vi "RxPkt - Init Packet Page.vi"(7 "Rx Section Cluster In":T2, 8 "error in (no error)":errorcluster, 11 "Node Ptr In":T1 format="%.0x") -> (0 "error out":errorcluster, 3 "Node Ptr Out":T1 format="%.0x", 5 "Rx Section Cluster Out":T2)   [LabVIEW 2016, in "UDP-Custom-Device System Explorer.lvlib"]
uses:
  UDP-Custom-Device System Explorer.lvlib
  Types/Page References/Refs - Rx Packets Page.ctl
  <vilib>/NI Veristand/Custom Device API/Custom Device Item Ref.ctl
  <vilib>/NI VeriStand/Custom Device API/Custom Device API.lvlib
  Property Accessors/Shared Packet Accessors.lvlib
  Property Accessors/Rx Channel Section Accessors.lvlib
  Property Accessors/Rx Packet Accessors.lvlib
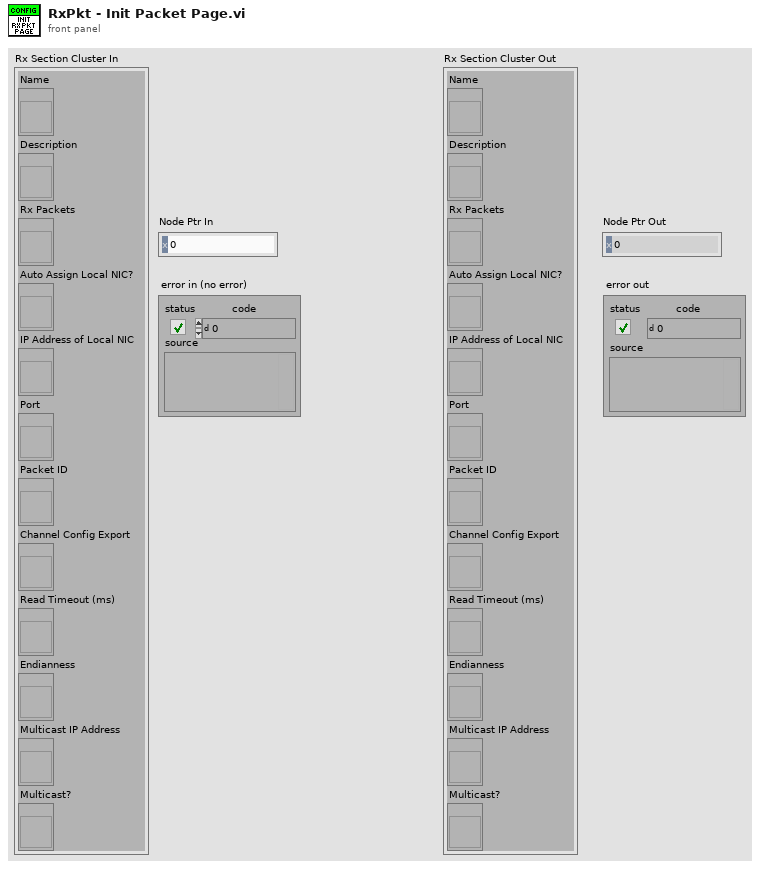
[diagram p1: front panel]
types:
  T1 = typedef "Custom Device API.lvlib/Custom Device Item Ref.ctl" = u64
  T2 = typedef "UDP-Custom-Device System Explorer.lvlib/Refs - Rx Packets Page.ctl" = cluster{"Name":refnum<vi>, "Description":refnum<vi>, "Rx Packets":refnum<vi>, "Auto Assign Local NIC?":refnum<vi>, "IP Address of Local NIC":refnum<vi>, "Port":refnum<vi>, "Packet ID":refnum<vi>, "Channel Config Export":refnum<vi>, "Read Timeout (ms)":refnum<vi>, "Endianness":refnum<vi>, "Multicast IP Address":refnum<vi>, "Multicast?":refnum<vi>}
  T3 = enum8{"Enabled", "Disabled", "Disabled and Grayed Out"}
  T4 = typedef "Custom Device API.lvlib/Custom Device Item Info.ctl" = cluster{"Name":string, "Is Channel":bool, "GUID":string, "Is Waveform":bool}
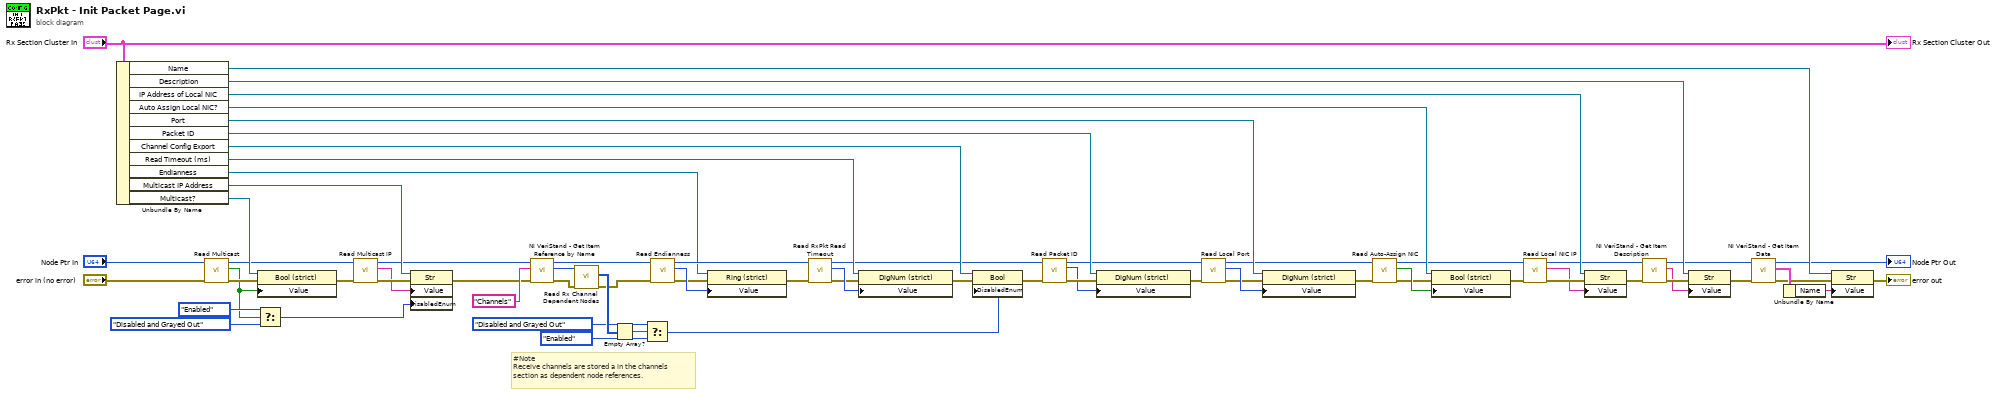
[diagram p0: block diagram]
diagram:
  # "#Note\nReceive channels are stored a in the channels\nsection as dependent node references."
  n1 = Unbundle By Name("Rx Section Cluster In") -> ("Name"=w65:refnum<vi>, "Description"=w64:refnum<vi>, "IP Address of Local NIC"=w54:refnum<vi>, "Auto Assign Local NIC?"=w55:refnum<vi>, "Port"=w66:refnum<vi>, "Packet ID"=w67:refnum<vi>, "Channel Config Export"=w37:refnum<vi>, "Read Timeout (ms)"=w27:refnum<vi>, "Endianness"=w19:refnum<vi>, "Multicast IP Address"=w13:refnum<vi>, "Multicast?"=w15:refnum<vi>)
  n2 = call "Read Multicast.vi"("error in (no error)"="error in (no error)", "Node Ptr"="Node Ptr In") -> ("error out"=w14:errorcluster, "Multicast"=w3:bool, "Node Ptr out"=w11:T1)  [unwired: 7 in]
  n3 = property class="Bool (strict)"(reference=w15, error in=w14, "Value"=w3) -> (error out=w9:errorcluster)  [unwired: 1 out]
  n4 = Select(t=T3."Enabled" ("Disabled"), s=w3, f=T3."Disabled and Grayed Out" ("Disabled")) -> (s? t:f=w4:T3)
  n5 = call "Read Multicast IP.vi"("error in (no error)"=w9, "Node Ptr"=w11) -> ("error out"=w8:errorcluster, "Multicast IP Address"=w7:string, "Node Ptr out"=w10:T1)  [unwired: 7 in]
  n6 = property class="Str"(reference=w13, error in=w8, "Value"=w7, "DisabledEnum"=w4) -> (error out=w12:errorcluster)  [unwired: 1 out]
  n7 = call <vilib>:"NI VeriStand - Get Item Reference by Name.vi"("error in (no error)"=w12, "Item Name"="Channels" ("Section Name"), "Parent Ref in"=w10) -> ("error out"=w33:errorcluster, "Item Ref"=w34:T1, "Parent Ref out"=w22:T1)  [unwired: 5 in, 1 out]
  n8 = call "Read Rx Channel Dependent Nodes.vi"("error in (no error)"=w33, "Node Ptr"=w34) -> ("error out"=w20:errorcluster, "Dependent Node Refs"=w32:T1[])  [unwired: 7 in, 1 out]
  n9 = Empty Array?(array=w32) -> (empty?=w29:bool)
  n10 = Select(t=T3."Disabled and Grayed Out" ("Disabled"), s=w29, f=T3."Enabled" ("Disabled")) -> (s? t:f=w28:T3)
  n11 = call "Read Endianness.vi"("error in (no error)"=w20, "Node Ptr"=w22) -> ("error out"=w17:errorcluster, "Endianness"=w18:u16, "Node Ptr out"=w21:T1)  [unwired: 7 in]
  n12 = property class="Ring (strict)"(reference=w19, error in=w17, "Value"=w18) -> (error out=w16:errorcluster)  [unwired: 1 out]
  n13 = call "Read RxPkt Read Timeout.vi"("error in (no error)"=w16, "Node Ptr"=w21) -> ("error out"=w24:errorcluster, "Read Timeout"=w26:i32, "Node Ptr out"=w25:T1)  [unwired: 7 in]
  n14 = property class="DigNum (strict)"(reference=w27, error in=w24, "Value"=w26) -> (error out=w23:errorcluster)  [unwired: 1 out]
  n15 = property class="Bool"(reference=w37, error in=w23, "DisabledEnum"=w28) -> (error out=w36:errorcluster)  [unwired: 1 out]
  n16 = call "Read Packet ID.vi"("error in (no error)"=w36, "Node Ptr"=w25) -> ("error out"=w52:errorcluster, "Packet ID"=w51:i32, "Node Ptr out"=w50:T1)  [unwired: 7 in]
  n17 = property class="DigNum (strict)"(reference=w67, error in=w52, "Value"=w51) -> (error out=w49:errorcluster)  [unwired: 1 out]
  n18 = call "Read Local Port.vi"("error in (no error)"=w49, "Node Ptr"=w50) -> ("error out"=w47:errorcluster, "Port"=w48:u16, "Node Ptr out"=w46:T1)  [unwired: 7 in]
  n19 = property class="DigNum (strict)"(reference=w66, error in=w47, "Value"=w48) -> (error out=w44:errorcluster)  [unwired: 1 out]
  n20 = call "Read Auto-Assign NIC.vi"("error in (no error)"=w44, "Node Ptr"=w46) -> ("error out"=w43:errorcluster, "Auto-Assign NIC"=w45:bool, "Node Ptr out"=w42:T1)  [unwired: 7 in]
  n21 = property class="Bool (strict)"(reference=w55, error in=w43, "Value"=w45) -> (error out=w41:errorcluster)  [unwired: 1 out]
  n22 = call "Read Local NIC IP.vi"("error in (no error)"=w41, "Node Ptr"=w42) -> ("error out"=w40:errorcluster, "IP Address of Local NIC"=w38:string, "Node Ptr out"=w39:T1)  [unwired: 7 in]
  n23 = property class="Str"(reference=w54, error in=w40, "Value"=w38) -> (error out=w53:errorcluster)  [unwired: 1 out]
  n24 = call <vilib>:"NI VeriStand - Get Item Description.vi"("error in (no error)"=w53, "Item Ref in"=w39) -> ("error out"=w63:errorcluster, "Description"=w62:string, "Item Ref out"=w60:T1)  [unwired: 7 out]
  n25 = property class="Str"(reference=w64, error in=w63, "Value"=w62) -> (error out=w61:errorcluster)  [unwired: 1 out]
  n26 = call <vilib>:"NI VeriStand - Get Item Data.vi"("error in (no error)"=w61, "Item Ref in"=w60) -> ("error out"=w68:errorcluster, "Item Info"=w69:T4, "Item Ref out"=→"Node Ptr Out":T1)  [unwired: 6 in, 1 out]
  n27 = Unbundle By Name(w69) -> ("Name"=w59:string)
  n28 = property class="Str"(reference=w65, error in=w68, "Value"=w59) -> (error out=→"error out":errorcluster)  [unwired: 1 out]
  "Rx Section Cluster Out" <- "Rx Section Cluster In"
